vi "DHE_SetArtifPatterns.vi"(2 "DHE_ArtifPatterns":string) -> ()   [LabVIEW 2016]
uses:
  private/vis/DHE_VarAction.ctl
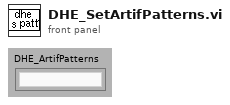
[diagram p1: front panel]
types:
  T1 = typedef "DHE_VarAction.ctl" = enum16{"read", "write"}
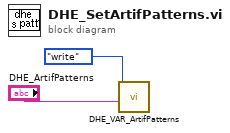
[diagram p0: block diagram]
diagram:
  n1 = call "DHE_VAR_ArtifPatterns.vi"("value"="DHE_ArtifPatterns", "action"=DHE_VarAction."write") -> ()  [unwired: 10 out]
